vi "Copy.vi"(5 "XRef":refnum<vi>, 6 "State In":T1={"Enum Type"=variant(dbl 0.0), "Types Type"=variant, "Enum Names"=[], "Type Names"=[], "Typedef Name"="", "Typedef Path"=path ""}) -> (0 "Reply":string[](array[string]), 2 "State Out":T1={"Enum Type"=variant(dbl 0.0), "Types Type"=variant, "Enum Names"=[], "Type Names"=[], "Typedef Name"="", "Typedef Path"=path ""})   [LabVIEW 2015, in "Define-Tagged-Union.xnode"]
doc: "This ability VI is called by LabVIEW after the user copies an XNode. State In is the same as the original XNode's state. The generated code is copied from the old XNode and will not be regenerated unless you return the GenerateCode reply.\n\nDefault behavior: Produce an exact copy of the original XNode without regenerating the code.\n\nThis ability does not provide UI and OS messages are not handled.\n\nSee also: Initialize"
uses:
  Define-Tagged-Union.xnode
  State.ctl
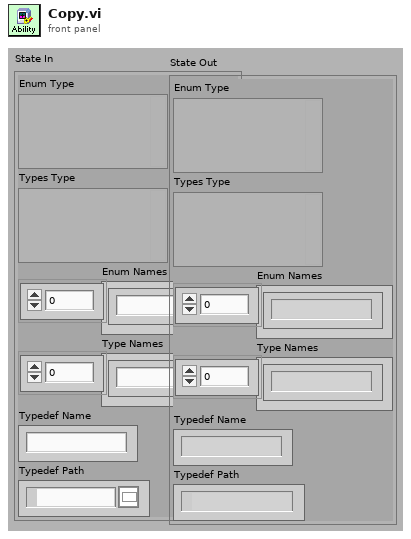
[diagram p1: front panel]
types:
  T1 = typedef "Define-Tagged-Union.xnode/State.ctl" = cluster{"Enum Type":variant, "Types Type":variant, "Enum Names":string[], "Type Names":string[], "Typedef Name":string, "Typedef Path":path}
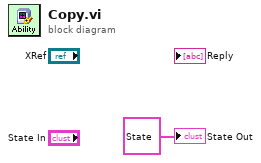
[diagram p0: block diagram]
diagram:
  "State Out" <- T1 {"Enum Type"=variant, "Types Type"=variant, "Enum Names"=[], "Type Names"=[], "Typedef Name"="", "Typedef Path"=path ""} ("State")
